vi "XIPIN_AXI_Chipscope_Monitor_3_05_a.vi"   [LabVIEW 2017]
doc: "This IP allows the user to tap the AXI signals from a design and observ these signal in analyzer for debug purpose.\n------------------------------------\n<b>Need License</b> : No"
uses:
  <vilib>/rvi/XilinxIP/XIPIN_XNode/niFpgaXIPIN.xnode
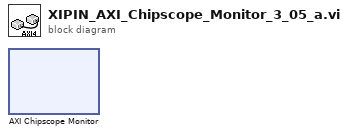
[diagram p0: block diagram]
diagram:
  n1 = xnode ("AXI Chipscope Monitor")() -> ()
